vi "Write Digitiser Enqueuer.vi"(8 "error in (no error)":errorcluster, 10 "Actor Framework:Message Enqueuer":refnum<class "Message Enqueuer.lvclass">, 11 "EmulatorActor in":refnum<class "EmulatorActor.lvclass">) -> (0 "error out":errorcluster, 3 "EmulatorActor out":refnum<class "EmulatorActor.lvclass">)   [LabVIEW 2019, in "EmulatorActor.lvlib" / "EmulatorActor.lvclass"]
uses:
  EmulatorActor.lvclass
  <vilib>/ActorFramework/Message Enqueuer/Message Enqueuer.lvclass
  EmulatorActor.lvclass/EmulatorActor.ctl
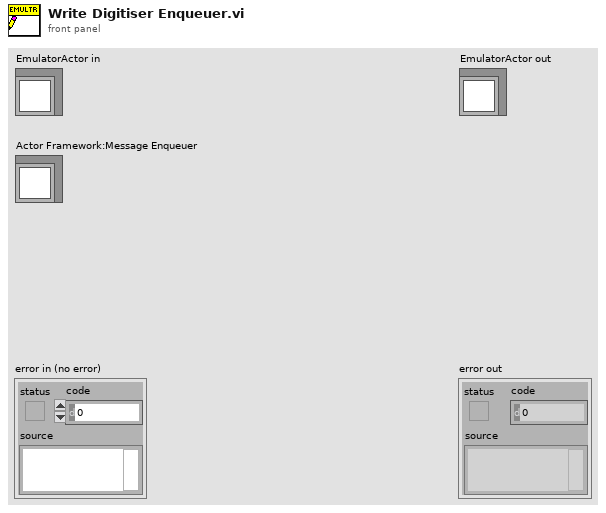
[diagram p1: front panel]
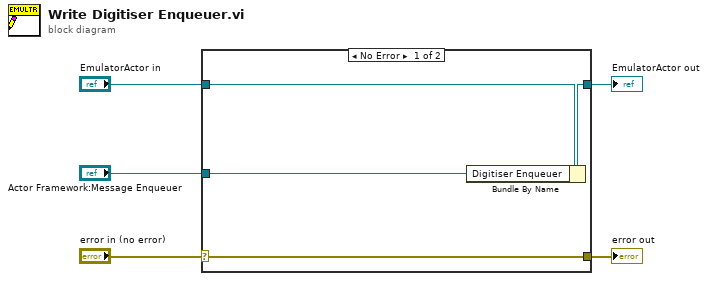
[diagram p0: block diagram]
diagram:
  n1 = case shown="No Error" "error in (no error)" {
    selector: "error in (no error)" -> [w9 w10]
    tunnel: [w9 w10] -> w4
    tunnel: [w7 w11] -> w2
    tunnel: "EmulatorActor in" -> [w8 w11]
    tunnel: "Actor Framework:Message Enqueuer" -> [w6 _]
    frame No Error {
      n2 = Bundle By Name(cluster=w8, "Digitiser Enqueuer"=w6) -> (w7:refnum<class "EmulatorActor.lvclass">)
    }
    frame Error {
    }
  }
  "error out" <- w4
  "EmulatorActor out" <- w2
